vi "215.Flush lines - cycles (SubVI).vi"(5 "Volume (uL)":i32=1000 min=0 max=1000 step=1, 7 "Syringe Cycle (ms)":u32=15000, 8 "Gilson 215 PORT":refnum<visa-resource-name>="COM12", 9 "VICI Multichannel valve":refnum<visa-resource-name>="COM12", 10 "Channel":i32=10 min=1 max=10 step=1, 11 "Cycles":i32=3 min=1 max=10 step=1) -> (0 "Gilson 215 PORT 2":refnum<visa-resource-name>="COM12", 1 "VICI Multichannel valve 2":refnum<visa-resource-name>="COM12", 3 "OK":bool)   [LabVIEW 2017]
panel:
  # "Channel 1 needle\nChannel 2 - loop 2\nChannel 3 - Loop 3\nChannel 4 - Loop 4\nChannel 10 - multichanel valve waste"
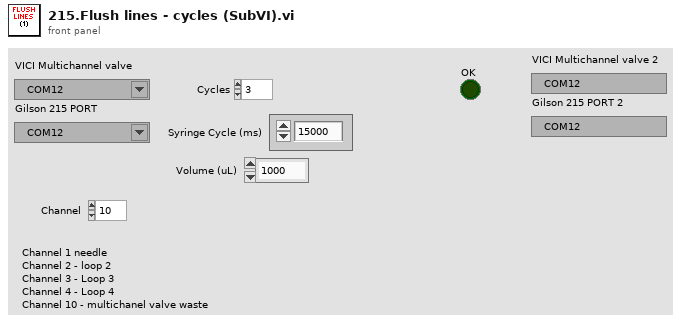
[diagram p1: front panel]
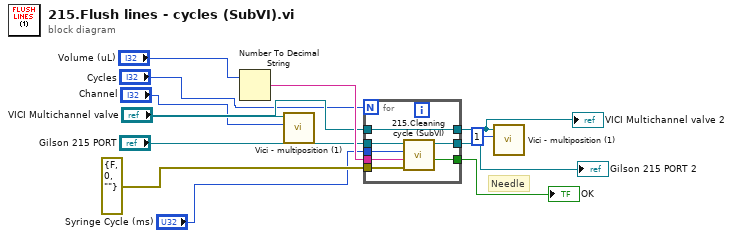
[diagram p0: block diagram]
diagram:
  # "Needle"
  n1 = Number To Decimal String(number="Volume (uL)") -> (decimal integer string=w11:string)  [unwired: 1 in]
  n2 = call "Vici - multiposition (1).vi"("Position"="Channel", "VISA resource name"="VICI Multichannel valve") -> ()  [unwired: 9 in, 1 out]
  n3 = for {
    N: "Cycles" -> [_]
    tunnel: "Gilson 215 PORT" -> [w19]
    tunnel: errorcluster {"status"=FALSE, "code"=0, "source"=""} ("error out") -> [w18]
    tunnel: w11 -> [w17]
    tunnel: [w16] -> w10
    tunnel: "Syringe Cycle (ms)" -> [w15]
    tunnel: "VICI Multichannel valve" -> [w14]
    tunnel: [w14] -> w2
    tunnel: [w13] -> w1
    n4 = call "215.Cleaning cycle (SubVI).vi"("error in (no error)"=w18, "Volumen (-1000 to 0)"=w17, "milliseconds to wait"=w15, "VISA Refnum in"=w19) -> ("Boolean"=w16:bool, "VISA out"=w13:refnum<visa-resource-name>)  [unwired: 5 in, 1 out]
  }
  "OK" <- w10
  "VICI Multichannel valve 2" <- w2
  "Gilson 215 PORT 2" <- w1
  n5 = call "Vici - multiposition (1).vi"("Position"=u32 1, "VISA resource name"=w2) -> ()  [unwired: 9 in, 1 out]
